vi "SingleEncoderData.vi"(6 "Reset?":bool=TRUE, 8 "Tick Constant":dbl, 10 "Rate":dbl, 11 "Distance":dbl) -> (3 "Encoder Data":T1 {"Ticks" format="%#.6g"})   [LabVIEW 2014]
uses:
  Common Code/Encoder Values.ctl
  <vilib>/addons/control/pid/NI_PID_pid.lvlib
  <vilib>/addons/control/pid/pid.llb/PID Control Input Filter (DBL).vi
panel:
  in  "Encoder Values TD":T1 {"Ticks" format="%#.6g"}
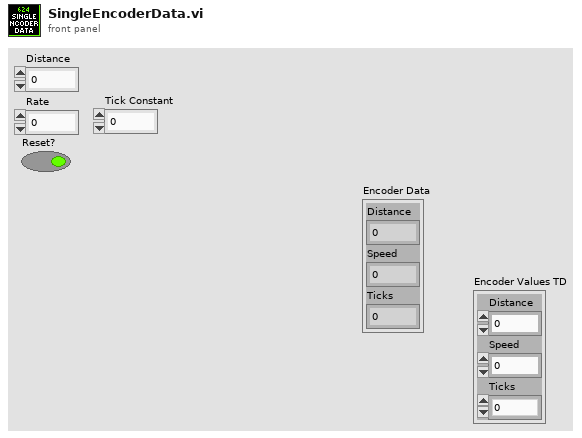
[diagram p1: front panel]
types:
  T1 = typedef "Encoder Values.ctl" = cluster{"Distance":dbl, "Speed":dbl, "Ticks":dbl}
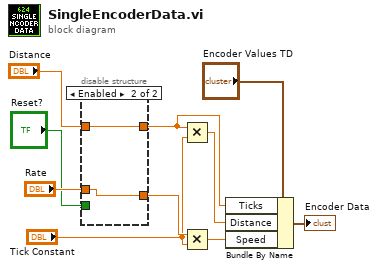
[diagram p0: block diagram]
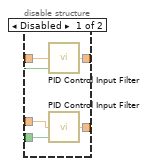
[diagram p2: hidden frame]
diagram:
  n1 = disable-structure shown="Enabled" {
    disable-tunnel: [w15 w16] -> w10
    disable-tunnel: "Distance" -> [w14 w17]
    disable-tunnel: "Rate" -> [w13 w16]
    disable-tunnel: "Reset?" -> [w12 _]
    disable-tunnel: [w11 w17] -> w1
    frame Disabled {
      n2 = call-poly <vilib>:"PID Control Input Filter.vi"("reinitialize? (F)"=w12, "input"=w14) -> ("output"=w11:dbl)  [unwired: 3 in]
      n3 = call-poly <vilib>:"PID Control Input Filter.vi"("reinitialize? (F)"=w12, "input"=w13) -> ("output"=w15:dbl)  [unwired: 3 in]
    }
    frame Enabled {
    }
  }
  n4 = Multiply(x=w1, y="Tick Constant") -> (x*y=w5:dbl)
  n5 = Multiply(x=w10, y="Tick Constant") -> (x*y=w4:dbl)
  n6 = Bundle By Name(cluster="Encoder Values TD", "Ticks"=w1, "Distance"=w5, "Speed"=w4) -> (→"Encoder Data":T1)
